vi "[FGV]Button Click Frequency.vi"(8 "error in (no error)":errorcluster, 11 "Command":enum16{"Initialize", "Add", "Read"}(ring)) -> (0 "error out":errorcluster, 3 "Value":i32)   [LabVIEW 2019]
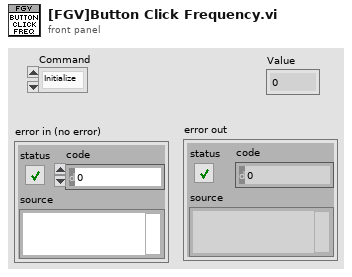
[diagram p1: front panel]
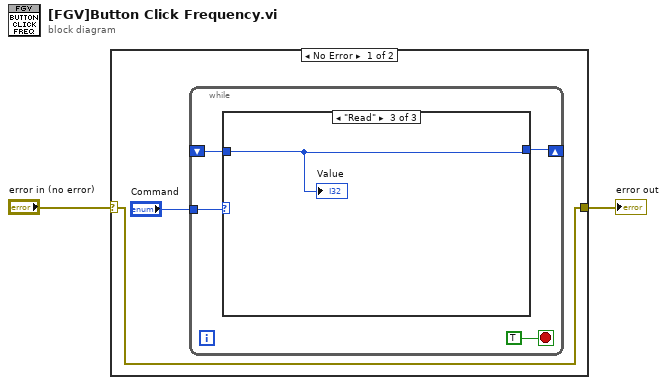
[diagram p0: block diagram]
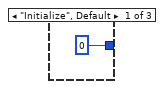
[diagram p2: hidden frame]
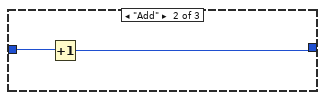
[diagram p3: hidden frame]
diagram:
  n1 = case shown="No Error" "error in (no error)" {
    selector: "error in (no error)" -> [w3 w13]
    tunnel: [w3 w13] -> w1
    frame No Error {
      n2 = while {
        tunnel: "Command" -> [w8]
        shift-right: [w6] -> _
        shift-left: _ -> [w5]
        stop <- TRUE stop-if-true
        n3 = case shown="\"Read\"" w8 {
          tunnel: [0 w10 w12] -> w6
          tunnel: w5 -> [_ w11 w12]
          frame "Initialize", Default {
          }
          frame "Add" {
            n4 = Increment(x=w11) -> (x+1=w10:i32)
          }
          frame "Read" {
            "Value" <- w12
          }
        }
      }
    }
    frame Error {
    }
  }
  "error out" <- w1
